vi "EXAMPLE APPLICATION.vi"() -> ()   [LabVIEW 2021]
uses:
  <vilib>/Instr/_visa.llb/VISA Configure Serial Port (Instr).vi
panel:
  in  "EMERGENCY":bool
  in  "Slide":u8(slide) scale=0.0..255.0
  out "Slide MCU Response":dbl(knob) scale=0.0..255.0
  out "Written?":bool
  out "Data to Send":i32[](array[numeric])
  out "(hi.lo)":u16
  out "Potentiometer:":dbl(knob) scale=0.0..1023.0
  in  "Start":bool
  in  "Write?":bool
  out "DBarray":dbl[][](array[numeric])
  in  "DB File":string="cansart_db.h"
  in  "stop":bool
  in  "BaudRate:":u32=115200
  in  "COM:":refnum<visa-resource-name>
  # "Cansart Example Application"
  # "Test Potentiometer by connecting a potentiometer\non the pin referred on your controller example"
  # "Double Click on the 1023 number to change it \nto a higher number depending on what your \nADC resolution"
  # "Engineered and Maintained by:\nGuilherme Candido\nteoriaeletrica@gmail.com"
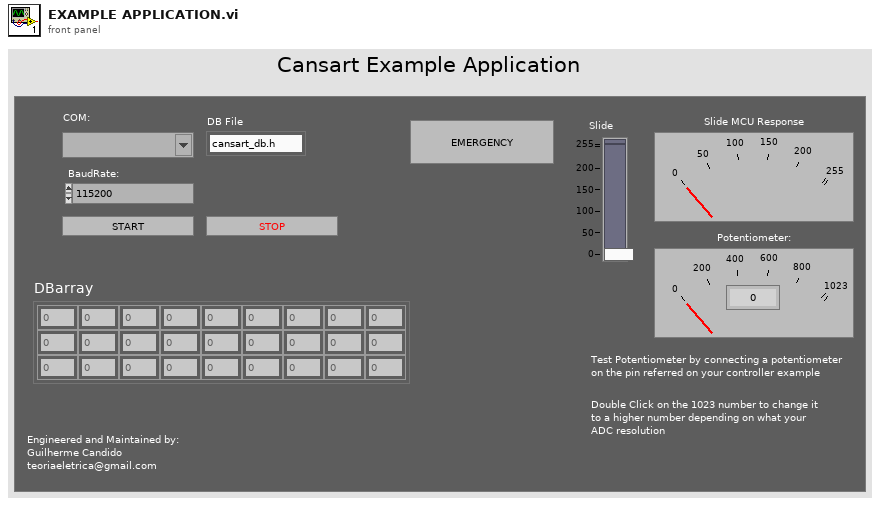
[diagram p1: front panel]
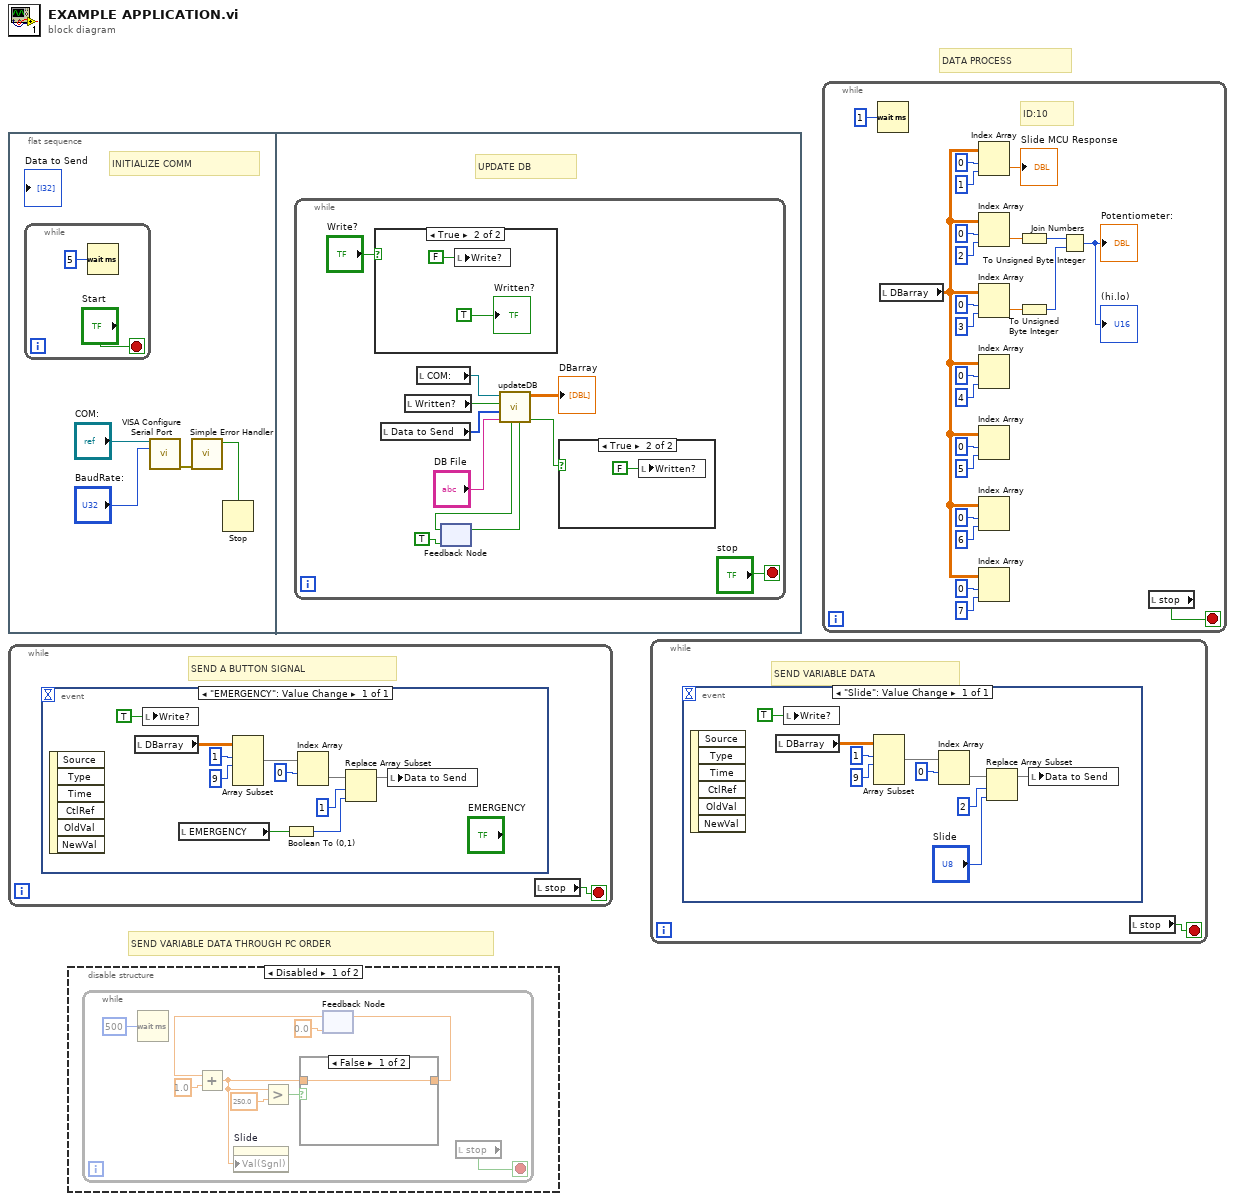
[diagram p0: block diagram]
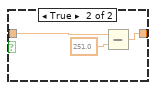
[diagram p2: hidden frame]
diagram:
  # "DATA PROCESS"
  # "SEND VARIABLE DATA THROUGH PC ORDER"
  n1 = flat-sequence {
    frame #0 {
      # "INITIALIZE COMM"
      n2 = while {
        stop <- "Start" stop-if-true
        n3 = Wait (ms)(milliseconds to wait=u32 5) -> ()  [unwired: 1 out]
      }
      n4 = call-poly "VISA Configure Serial Port"("VISA resource name"="COM:", "baud rate (9600)"="BaudRate:") -> ("error out"=w2:errorcluster)  [unwired: 12 in, 1 out]
      n5 = call <vilib>:"Simple Error Handler.vi"("error in (no error)"=w2) -> ("error?"=w1:bool)  [unwired: 4 in, 4 out]
      n6 = Stop(stop? (T)=w1) -> ()
    }
    frame #1 {
      # "UPDATE DB"
      n7 = while {
        stop <- "stop" stop-if-true
        n8 = case shown="True" "Write?" {
          frame False {
          }
          frame True {
            n9 = local write "Write?"(FALSE ("Write?")) -> ()
            "Written?" <- TRUE ("Boolean")
          }
        }
        n10 = local read "Data to Send"() -> (w12:i32[])
        n11 = local read "Written?"() -> (w9:bool)
        n12 = local read "COM:"() -> (w16:refnum<visa-resource-name>)
        n13 = feedback #1(TRUE ("First 2")) -> (w8:bool)
        n14 = call "updateDB.vi"("First"=w8, "DBname"="DB File", "Data Write"=w12, "Write?"=w9, "COM PORT"=w16) -> ("Written!"=w10:bool, "DBarray"=→"DBarray":dbl[][], "First 2"=w7:bool)  [unwired: 4 in]
        n15 = feedback-in #1(w7) -> ()
        n16 = case shown="True" w10 {
          frame False {
          }
          frame True {
            n17 = local write "Written?"(FALSE ("Written?")) -> ()
          }
        }
      }
    }
  }
  n18 = while {
    stop <- w21 stop-if-true
    # "SEND A BUTTON SIGNAL"
    n19 = event shown="[0] \"EMERGENCY\": Value Change" {
      selector: _ -> [_]
      dyn-events: _ -> [_]
      timeout: _ -> [_]
      event "EMERGENCY": Value Change {
        n20 = event-data() -> ()  [unwired: 1 in, 6 out]
        n21 = local read "DBarray"() -> (w28:dbl[][])
        n22 = local write "Write?"(TRUE ("Write?")) -> ()
        n23 = local read "EMERGENCY"() -> (w31:bool)
        n24 = Array Subset(array=w28, index (row)=1 ("index"), length (row)=9 ("length")) -> (w27:dbl[][])  [unwired: 2 in]
        n25 = Boolean To (0,1)(Boolean=w31) -> (0, 1=w22:i16)
        n26 = Index Array(array=w27, index (row)=0) -> (element=w29:dbl[])  [unwired: 1 in]
        n27 = Replace Array Subset(array=w29, new element=w22, index=1) -> (w30:dbl[])
        n28 = local write "Data to Send"(w30) -> ()
      }
    }
    n29 = local read "stop"() -> (w21:bool)
  }
  n30 = disable-structure shown="Disabled" {
    frame Disabled {
      n31 = while {
        stop <- w41 stop-if-true
        n32 = Wait (ms)(milliseconds to wait=u32 500) -> ()  [unwired: 1 out]
        n33 = feedback #2(0.0) -> (w35:dbl)
        n34 = Add(x=w35, y=1.0) -> (x+y=w33:dbl)
        n35 = property on="Slide" class="Slide (strict)"("Val(Sgnl)"=w33) -> ()  [unwired: 2 in, 2 out]
        n36 = Greater?(x=w33, y=250.0) -> (0:w37:bool)
        n37 = case shown="False" w37 {
          tunnel: [w42 w44] -> w36
          tunnel: w33 -> [w42 w43]
          frame False {
          }
          frame True {
            n38 = Subtract(x=w43, y=251.0) -> (x-y=w44:dbl)
          }
        }
        n39 = feedback-in #2(w36) -> ()
        n40 = local read "stop"() -> (w41:bool)
      }
    }
    frame Enabled {
    }
  }
  n41 = while {
    stop <- w46 stop-if-true
    # "SEND VARIABLE DATA"
    n42 = event shown="[0] \"Slide\": Value Change" {
      selector: _ -> [_]
      dyn-events: _ -> [_]
      timeout: _ -> [_]
      event "Slide": Value Change {
        n43 = event-data() -> ()  [unwired: 1 in, 6 out]
        n44 = local read "DBarray"() -> (w50:dbl[][])
        n45 = local write "Write?"(TRUE ("Write?")) -> ()
        n46 = Array Subset(array=w50, index (row)=1 ("index"), length (row)=9 ("length")) -> (w55:dbl[][])  [unwired: 2 in]
        n47 = Index Array(array=w55, index (row)=0) -> (element=w56:dbl[])  [unwired: 1 in]
        n48 = Replace Array Subset(array=w56, new element="Slide", index=2) -> (w48:dbl[])
        n49 = local write "Data to Send"(w48) -> ()
      }
    }
    n50 = local read "stop"() -> (w46:bool)
  }
  n51 = while {
    stop <- w69 stop-if-true
    # "ID:10"
    n52 = Wait (ms)(milliseconds to wait=u32 1) -> ()  [unwired: 1 out]
    n53 = local read "DBarray"() -> (w63:dbl[][])
    n54 = Index Array(array=w63, index (row)=0, index (col)=1 ("disabled index (col)")) -> (element=→"Slide MCU Response":dbl)
    n55 = Index Array(array=w63, index (row)=0 ("disabled index (row)"), index (col)=2 ("disabled index (col)")) -> (element=w75:dbl)
    n56 = Index Array(array=w63, index (row)=0 ("disabled index (row)"), index (col)=3 ("disabled index (col)")) -> (element=w78:dbl)
    n57 = Index Array(array=w63, index (row)=0 ("disabled index (row)"), index (col)=4 ("disabled index (col)")) -> ()  [unwired: 1 out]
    n58 = Index Array(array=w63, index (row)=0 ("disabled index (row)"), index (col)=5 ("disabled index (col)")) -> ()  [unwired: 1 out]
    n59 = Index Array(array=w63, index (row)=0 ("disabled index (row)"), index (col)=6 ("disabled index (col)")) -> ()  [unwired: 1 out]
    n60 = Index Array(array=w63, index (row)=0 ("disabled index (row)"), index (col)=7 ("disabled index (col)")) -> ()  [unwired: 1 out]
    n61 = To Unsigned Byte Integer(number=w75) -> (unsigned 8bit integer=w79:u8)
    n62 = To Unsigned Byte Integer(number=w78) -> (unsigned 8bit integer=w77:u8)
    n63 = Join Numbers(hi=w79, lo=w77) -> ((hi.lo)=→"(hi.lo)" →"Potentiometer:":u16)
    n64 = local read "stop"() -> (w69:bool)
  }
